vi "多参数全局变量.vi"() -> ()   [LabVIEW 2016, in "斯坦道多参数.lvlib"]
uses:
  <vilib>/Plasmionique/MB Master/MB_Master/MB_Master.lvclass
panel:
  in  "MB session in 电导率":refnum<class "MB_Master.lvclass">
  out "TCP Connection Count":u32
  out "远程校准运行状态":T1
  out "校准运行状态":T1
  in  "权限":enum16{"一级权限", "二级权限", "三级权限"}(ring)
  out "ORP显示":T2
  out "orp通讯状态":bool
  out "配置文件 path":path
  out "ping":bool
  out "副屏状态":u16(ring) items=["空闲", "水样测试", "标样核查", "停止"]
  out "主屏状态":u16(ring) items=["空闲", "水样测试", "标样核查", "停止"]
  in  "副屏IP":cluster{"address":string, "port (502)":u16}={"address"="192.168.1.101", "port (502)"=110}
  out "主副屏同步启动":u16(ring) items=["空闲", "水样测试", "标样核查", "停止"]
  in  "主屏IP":cluster{"address":string, "port (502)":u16}={"address"="192.168.1.100", "port (502)"=110}
  out "蓝绿藻通讯状态":bool
  out "藻密度通讯状态":bool
  out "叶绿素a通讯状态":bool
  out "浊度通讯状态":bool
  out "spcond通讯状态":bool
  out "DO通讯状态":bool
  out "ph通讯状态":bool
  in  "校准VI引用句柄":T3
  in  "MB session in":refnum<class "MB_Master.lvclass">
  in  "运行模式":enum16{"维护模式", "常规模式", "应急模式", "质控模式"}(ring)=enum."常规模式"
  in  "多参数编号":string
  out "藻密度显示":T2
  out "蓝绿藻显示":T2
  out "cond显示":T2
  out "盐度显示":T2
  out "spcond显示":T2
  out "ph显示":T2
  out "水温显示":T4={"CH"=1, "监测值"=0.0, "温度偏移修正值"=0.0, "信号值"=0.0} {"CH" items=["pH", "Cond", "DO", "Turb"]}
  out "浊度显示":T2
  out "DO显示":T5
  out "叶绿素a显示":T2
  out "多参数运行状态":u16(ring) items=["空闲", "水样测试", "标样核查"]
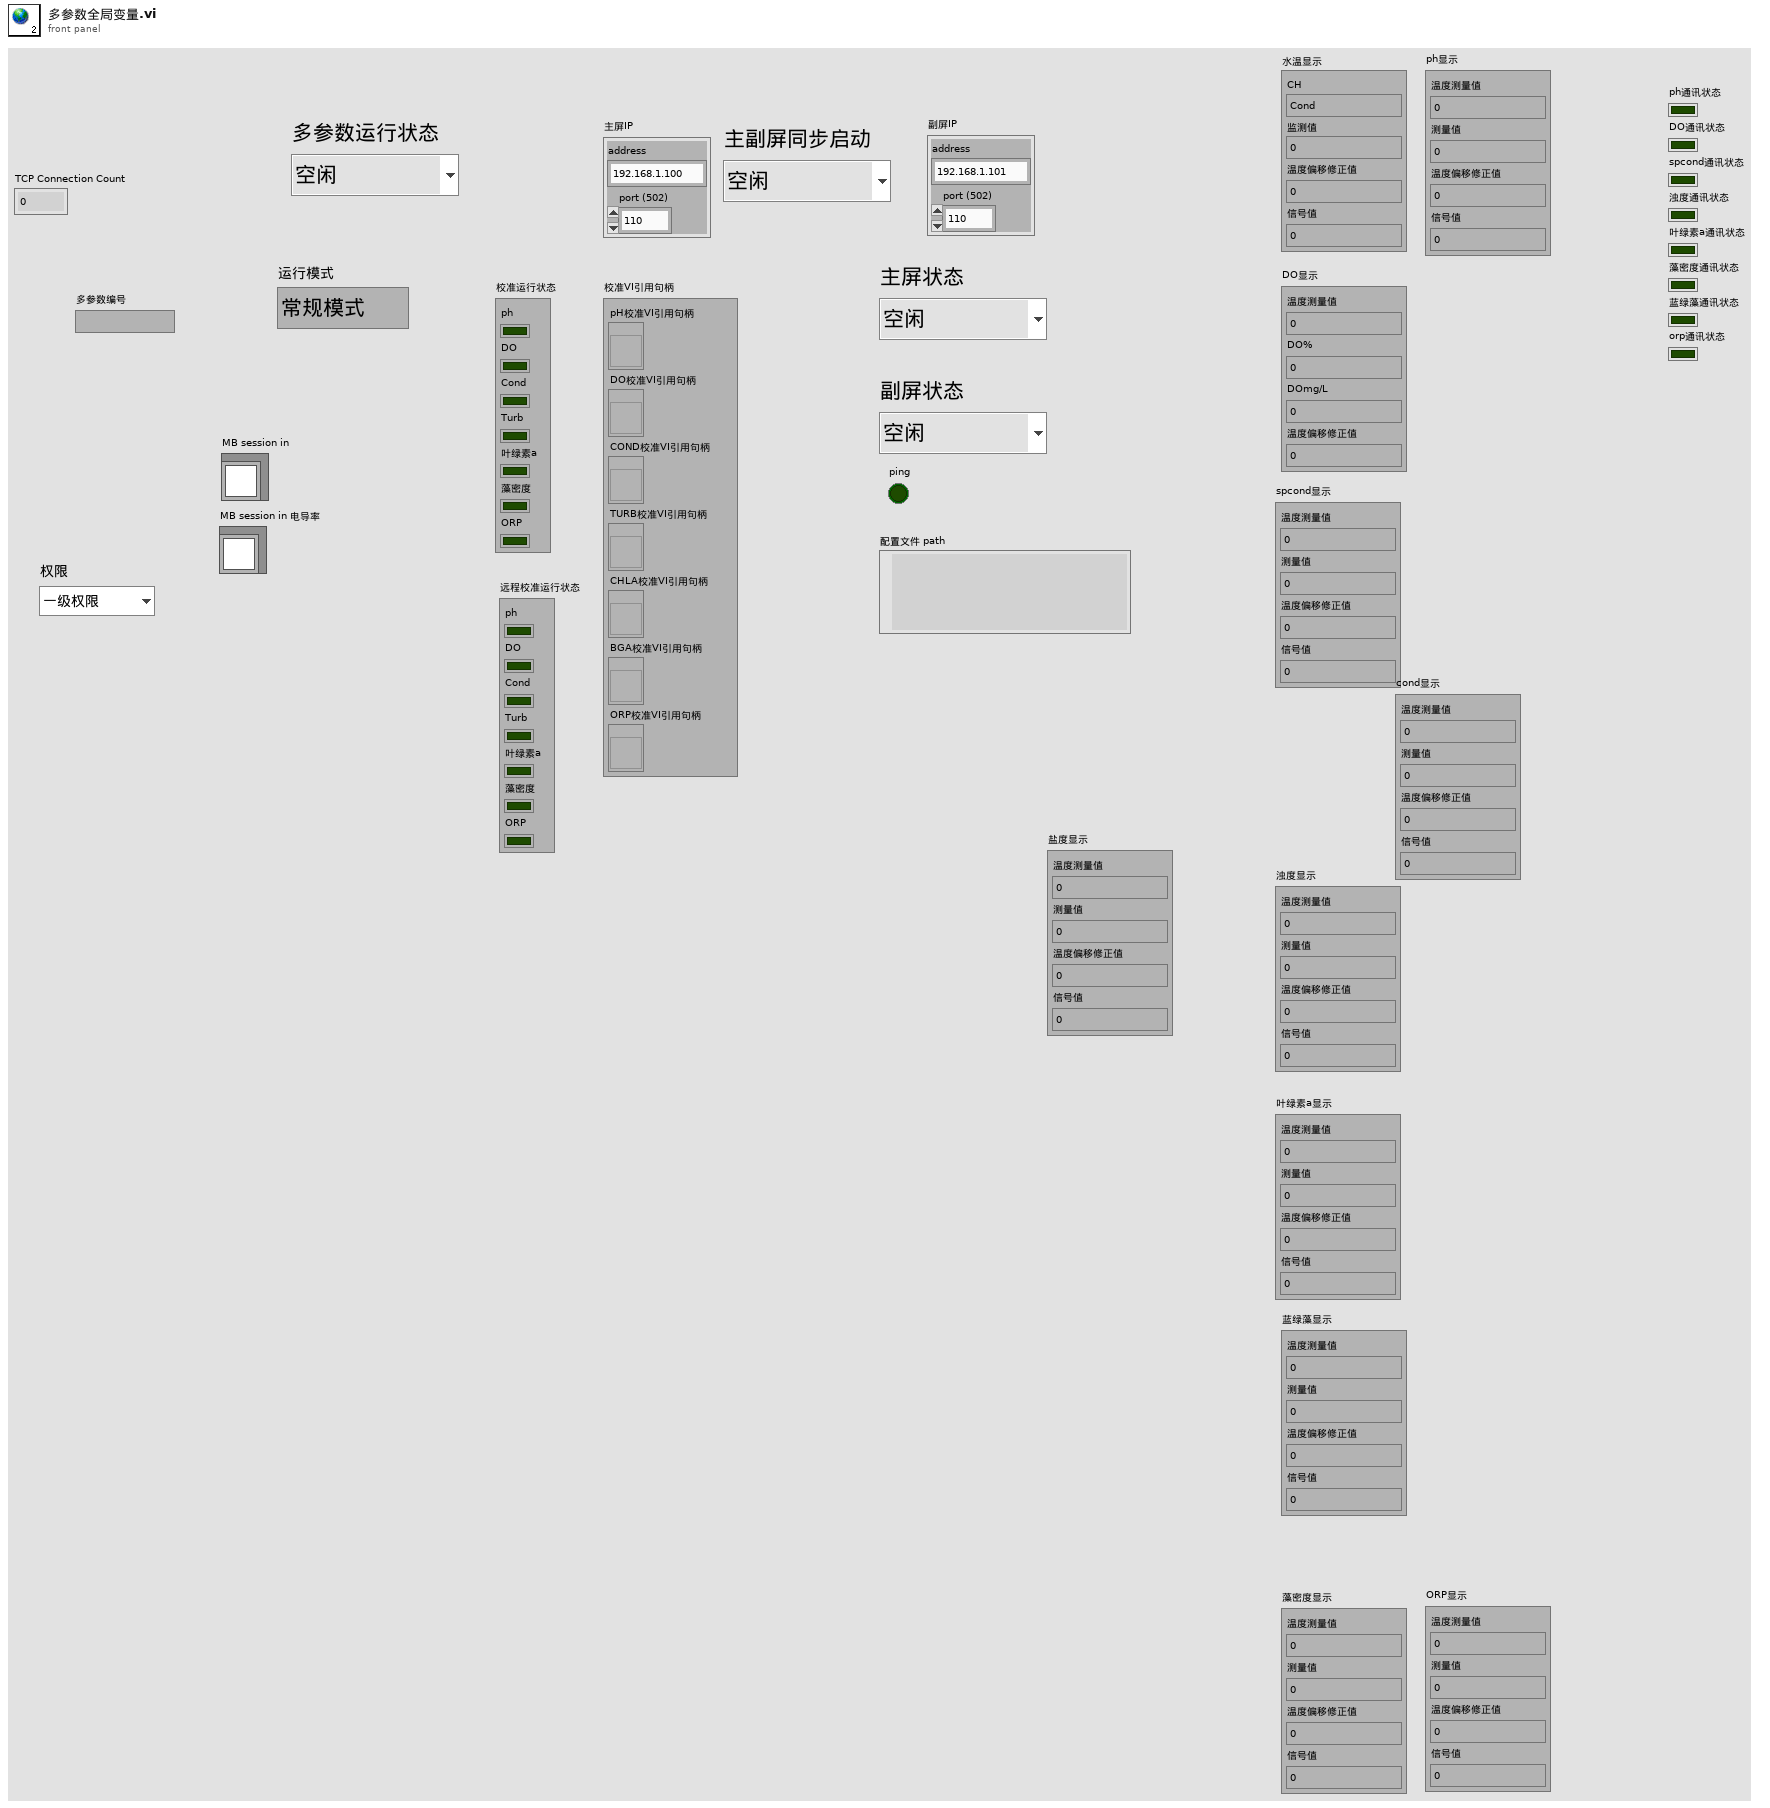
[diagram p1: front panel]
types:
  T1 = cluster{"ph":bool, "DO":bool, "Cond":bool, "Turb":bool, "叶绿素a":bool, "藻密度":bool, "ORP":bool}
  T2 = cluster{"温度测量值":sgl, "测量值":sgl, "温度偏移修正值":sgl, "信号值":sgl}
  T3 = cluster{"pH校准VI引用句柄":refnum<vi>, "DO校准VI引用句柄":refnum<vi>, "COND校准VI引用句柄":refnum<vi>, "TURB校准VI引用句柄":refnum<vi>, "CHLA校准VI引用句柄":refnum<vi>, "BGA校准VI引用句柄":refnum<vi>, "ORP校准VI引用句柄":refnum<vi>}
  T4 = cluster{"CH":u16, "监测值":dbl, "温度偏移修正值":sgl, "信号值":sgl}
  T5 = cluster{"温度测量值":sgl, "DO%":sgl, "DOmg/L":sgl, "温度偏移修正值":sgl}
diagram:
